vi "main.vi"() -> ()   [LabVIEW 2019]
panel:
  in  "Timer (Stunde)":dbl
  out "Cold Plate":dbl(graph)
  out "Sample Plate":dbl(graph)
  out "Cold Plate Temperature":dbl
  in  "Stopp":bool
  in  "Sample":dbl
  in  "Cold Plate":dbl
  out "Sample Temperature":dbl
  out "AttoDryCode":path
  out "Status":dbl
  # "Input"
  # "Während des Tests"
  # "Temperaturen"
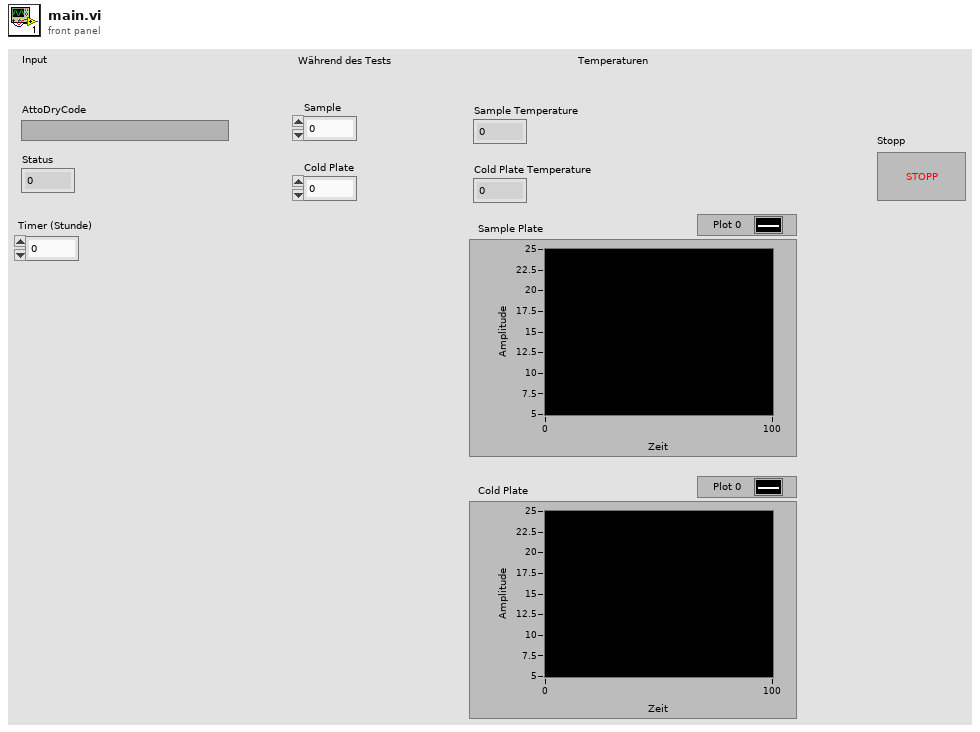
[diagram p1: front panel]
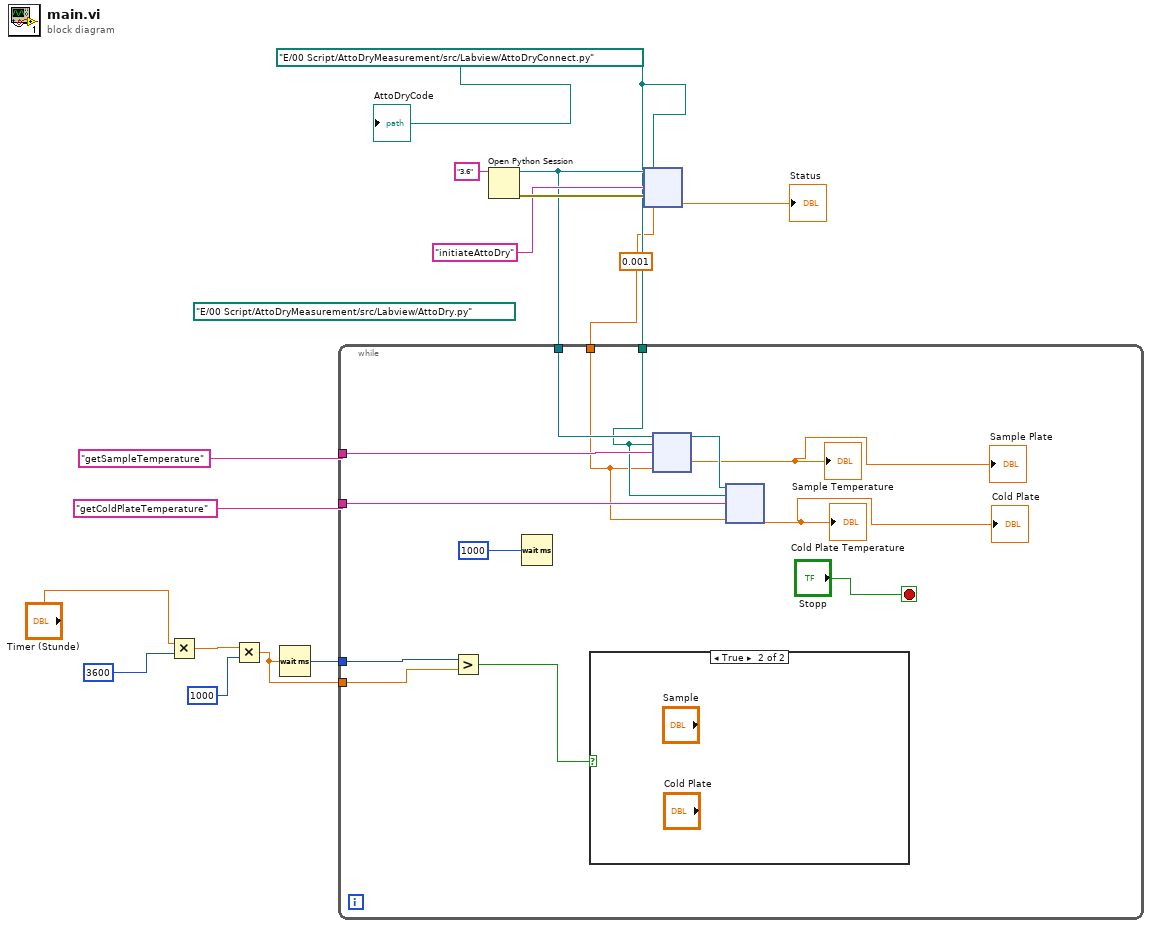
[diagram p0: block diagram]
diagram:
  w8 = 0.001
  (unwired) path "E:/00 Script/AttoDryMeasurement/src/Labview/AttoDry.py" ("Pfad")
  w10 = path "E:/00 Script/AttoDryMeasurement/src/Labview/AttoDryConnect.py" ("Pfad")
  n1 = Multiply(x="Timer (Stunde)", y=u32 3600 ("Zu wartende ms")) -> (x*y=w4:dbl)
  n2 = Multiply(x=w4, y=u32 1000 ("Zu wartende ms")) -> (x*y=w2:dbl)
  n3 = Wait (ms)(milliseconds to wait=w2) -> (millisecond timer value=w6:u32)
  n4 = Open Python Session(python version="3.6" ("Python-Version")) -> (session out=w11:refnum<k35>, error out=w15:errorcluster)  [unwired: 2 in]
  n5 = while {
    tunnel: w11 -> [w28]
    tunnel: w10 -> [w23]
    tunnel: "getSampleTemperature" ("Funktionsname") -> [w27]
    tunnel: w8 -> [w21]
    tunnel: "getColdPlateTemperature" ("Funktionsname") -> [w22]
    tunnel: w6 -> [w18]
    tunnel: w2 -> [w16]
    stop <- "Stopp" stop-if-true
    n6 = Greater?(x=w18, y=w16) -> (0:w17:bool)
    n7 = Wait (ms)(milliseconds to wait=u32 1000 ("Zu wartende ms")) -> ()  [unwired: 1 out]
    n8 = case shown="True" w17 {
      frame False {
      }
      frame True {
      }
    }
    n9 = node(w28, w23, w27, w21) -> (w24:refnum<k35>, →"Sample Temperature" →"Sample Plate":dbl)  [unwired: 1 in, 3 out]
    n10 = node(w24, w23, w22, w21) -> (→"Cold Plate Temperature" →"Cold Plate":dbl)  [unwired: 1 in, 4 out]
  }
  n11 = node(w11, w10, "initiateAttoDry" ("Funktionsname"), w15, w8) -> (→"Status":dbl)  [unwired: 4 out]
  "AttoDryCode" <- w10
